vi "Run.vi"(9 "Team in":refnum<class "Team.lvclass">, 11 "MySquare in":refnum<class "MySquare.lvclass">) -> (1 "Team out":refnum<class "Team.lvclass">, 2 "Run Result":T1, 3 "Square out":refnum<class "Square.lvclass">)   [LabVIEW 2020, in "DemoTeam.lvlib" / "MySquare.lvclass"]
doc: "This VI is called on every active square each turn of the game for the square to decide what action to take."
uses:
  MySquare.lvclass
  C:/dev/lv20CE/sol-squarebattle/ProjectTemplates/Source/SummerOfLabVIEW/SquareBattle/template/SquareBattle/Square/Square.lvclass
  SquareBattle/Run Result.ctl
  SquareBattle/Square/Square.lvclass
  SquareBattle/Action.ctl
  SquareBattle/Direction.ctl
  SquareBattle/Team/Team.lvclass
  MyTeam/MyTeam.lvclass
  C:/dev/lv20CE/sol-squarebattle/ProjectTemplates/Source/SummerOfLabVIEW/SquareBattle/template/SquareBattle/Team/Team.lvclass
  SquareBattle/Square/Square.lvclass/Square.ctl
  <vilib>/numeric/Random Number (Range) U64.vi
  <vilib>/numeric/sub_Random U32.vi
  MySquare.lvclass/MySquare.ctl
  SquareBattle/SquareBattle.lvlib
  C:/dev/lv20CE/sol-squarebattle/ProjectTemplates/Source/SummerOfLabVIEW/SquareBattle/template/Squares/Demo/SquareTeam/MySquare/MySquare.lvclass
  C:/dev/lv20CE/sol-squarebattle/ProjectTemplates/Source/SummerOfLabVIEW/SquareBattle/template/Squares/Demo/SquareTeam/MyTeam/MyTeam.lvclass
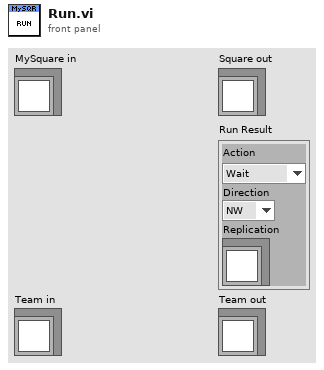
[diagram p1: front panel]
types:
  T1 = typedef "SquareBattle.lvlib/Run Result.ctl" = cluster{"Action":T2, "Direction":T3, "Replication":refnum<class "Square.lvclass">}
  T2 = typedef "SquareBattle.lvlib/Action.ctl" = enum16{"Wait", "Move", "Attack", "Replicate"}
  T3 = typedef "SquareBattle.lvlib/Direction.ctl" = enum16{"NW", "N", "NE", "E", "SE", "S", "SW", "W"}
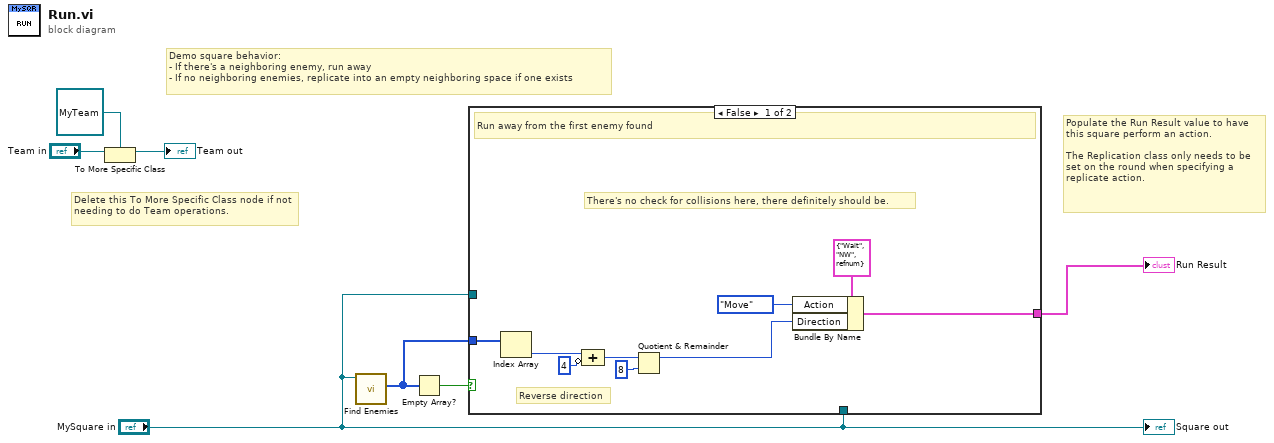
[diagram p0: block diagram]
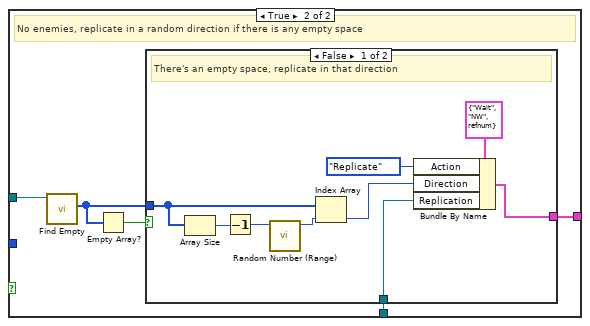
[diagram p2: hidden frame]
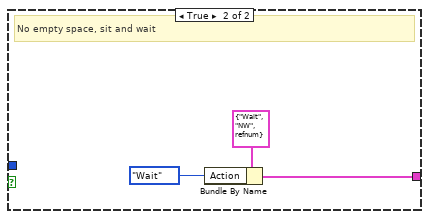
[diagram p3: hidden frame]
diagram:
  # "Demo square behavior:\n- If there's a neighboring enemy, run away\n- If no neighboring enemies, replicate into an empty neighboring space if one exists"
  # "Populate the Run Result value to have this square perform an action.\n\nThe Replication class only needs to be set on the round when specifying a replicate action."
  # "Delete this To More Specific Class node if not needing to do Team operations."
  n1 = To More Specific Class(target class=refnum<class "MyTeam.lvclass"> refnum ("SquareTeam.lvlib:MyTeam.lvclass"), reference="Team in") -> (specific class reference=→"Team out":refnum<class "MyTeam.lvclass">)  [unwired: 1 in, 1 out]
  n2 = call "Find Enemies.vi"("Square"="MySquare in") -> ("Enemy Directions"=w3:T3[])  [unwired: 10 in]
  n3 = Empty Array?(array=w3) -> (empty?=w4:bool)
  n4 = case shown="False" w4 {
    tunnel: w3 -> [w16 _]
    tunnel: [w13 w18] -> w2
    tunnel: "MySquare in" -> [_ w21]
    tunnel: "MySquare in" -> [_ w17]
    frame False {
      # "There's no check for collisions here, there definitely should be."
      # "Reverse direction"
      # "Run away from the first enemy found"
      n5 = Index Array(array=w16) -> (element=w9:T3)  [unwired: 1 in]
      n6 = Compound Arithmetic op=unknown(w9, invert 4 ("value")) -> (w11:i32)
      n7 = Quotient & Remainder(x=w11, y=8) -> (x-y*floor(x/y)=w8:i32)  [unwired: 1 out]
      n8 = Bundle By Name(cluster=T1 {"Action"=enum."Wait", "Direction"=enum."NW", "Replication"=refnum} ("Run Result"), "Action"=Action."Move", "Direction"=w8) -> (w13:T1)
    }
    frame True {
      # "No enemies, replicate in a random direction if there is any empty space"
      n9 = call "Find Empty.vi"("Square"=w21) -> ("Empty Directions"=w19:T3[])  [unwired: 10 in]
      n10 = Empty Array?(array=w19) -> (empty?=w20:bool)
      n11 = case shown="False" w20 {
        tunnel: w19 -> [w28 _]
        tunnel: [w22 w31] -> w18
        tunnel: w17 -> [w23 _]
        frame False {
          # "There's an empty space, replicate in that direction"
          n12 = Array Size(array=w28) -> (size(s)=w30:i32)
          n13 = Decrement(x=w30) -> (x-1=w29:i32)
          n14 = call-poly <vilib>:"Random Number (Range).vi"("upper bound (100)"=w29) -> ("number"=w27:u64)  [unwired: 10 in]
          n15 = Index Array(array=w28, index=w27) -> (element=w24:T3)
          n16 = Bundle By Name(cluster=T1 {"Action"=enum."Wait", "Direction"=enum."NW", "Replication"=refnum} ("Run Result"), "Action"=Action."Replicate", "Direction"=w24, "Replication"=w23) -> (w22:T1)
        }
        frame True {
          # "No empty space, sit and wait"
          n17 = Bundle By Name(cluster=T1 {"Action"=enum."Wait", "Direction"=enum."NW", "Replication"=refnum} ("Run Result"), "Action"=Action."Wait") -> (w31:T1)
        }
      }
    }
  }
  "Run Result" <- w2
  "Square out" <- "MySquare in"
